vi "Robot Global Data.vi"() -> ()   [LabVIEW 2014]
doc: "This global VI can contain as many global variables as you need. Place a control on the panel, give it a good name. To read or write to it from a VI, drag the icon to the diagram of that VI. You can also drag from the project. Click on the node to change which global you access. You shouldn't have multiple locations writing to a global or it will cause a race-condition."
uses:
  <vilib>/Rock Robotics/WPI/Camera/WPI_CameraImageSize.ctl
  <vilib>/Rock Robotics/WPI/DriverStation/WPI_DriverStationRobotMode2.ctl
panel:
  out "Drive: Front Right T":dbl
  out "Drive: Front Left T":dbl
  out "Drive: Rear Right T":dbl
  out "Drive: Rear Left T":dbl
  out "Gyro":dbl
  out "Detected Totes":T1(array[cluster]) {"Normalized Rect"."Numeric 5" format="%#_2g"; "Normalized Rect"."Numeric 3" format="%#_2g"; "Normalized Rect"."Numeric 2" format="%#_2g"; "Normalized Rect"."Numeric" format="%#_2g"}
  out "ms to process":dbl
  out "Talon 1":dbl
  out "Drive: Front Right":dbl
  out "Drive: Front Left":dbl
  out "Drive: Rear Right":dbl
  out "Drive: Rear Left":dbl
  out "PDP":dbl
  out "PCM":dbl
  in  "DriveRotation":dbl(slide) scale=-1.0..1.0
  in  "DriveY":dbl(slide) scale=-1.0..1.0
  in  "DriveX":dbl(slide) scale=-1.0..1.0
  in  "Axis 6":dbl(slide) scale=-1.0..1.0
  in  "Axis 5":dbl(slide) scale=-1.0..1.0
  in  "Axis 4":dbl(slide) scale=-1.0..1.0
  in  "Axis 3":dbl(slide) scale=-1.0..1.0
  in  "Axis 2":dbl(slide) scale=-1.0..1.0
  in  "Axis 1":dbl(slide) scale=-1.0..1.0
  out "Button 12":bool
  out "Button 11":bool
  out "Button 10":bool
  out "Button 9":bool
  out "Button 8":bool
  out "Button 7":bool
  out "Button 6":bool
  out "Button 5":bool
  out "Button 4":bool
  out "Button 3":bool
  out "Button 2":bool
  out "Button 1":bool
  in  "Robot Mode":T2
  in  "image size":T3=enum."320x240"
  in  "Enable Vision":bool
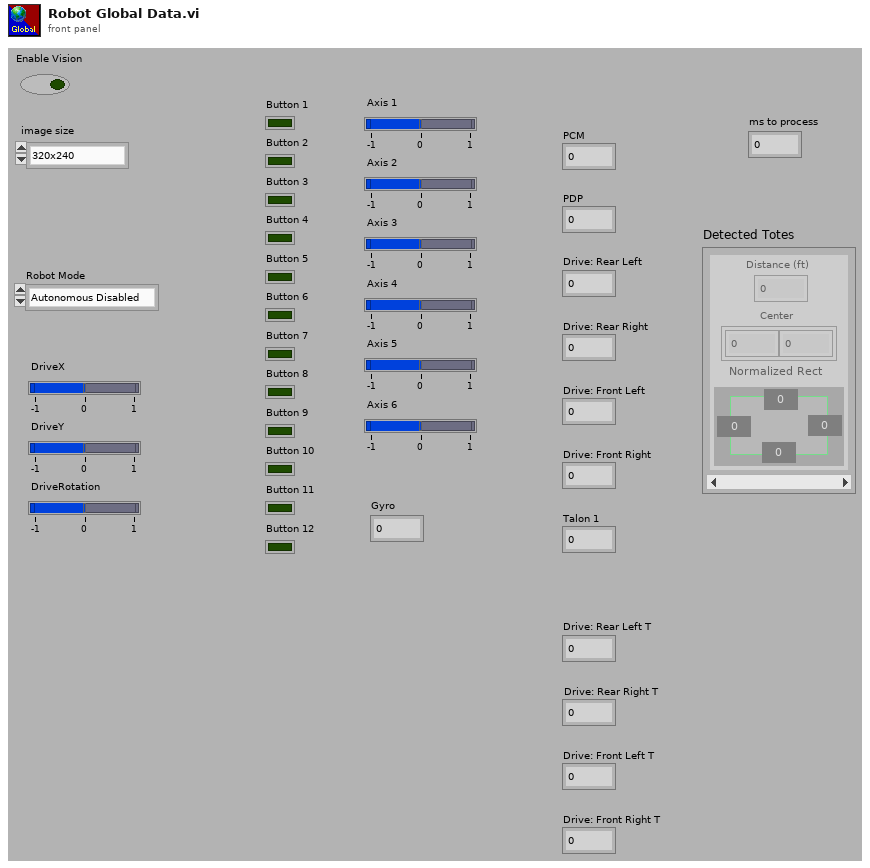
[diagram p1: front panel]
types:
  T1 = cluster{"Distance (ft)":dbl, "Center":cluster{dbl, dbl}, "Normalized Rect":cluster{"Numeric":dbl, "Numeric 2":dbl, "Numeric 3":dbl, "Numeric 5":dbl}}[]
  T2 = typedef "WPI_DriverStationRobotMode2.ctl" = enum16{"Autonomous Disabled", "Autonomous Enabled", "Teleop Disabled", "Teleop Enabled", "Disconnected", "Finish", "Test Disabled", "Test Enabled", "Emergency Stopped"}
  T3 = typedef "WPI_CameraImageSize.ctl" = enum16{"640x480", "320x240", "160x120", "Custom"}
diagram:
